vi "Vector Magnitude.vi"(1 "Z Component":dbl, 2 "Y Component":dbl, 3 "X Component":dbl) -> (0 "Magnitude":dbl)   [LabVIEW 2012]
doc: "Computes the magnitude of a two- or three-dimensional vector using the distance formula. For a two-dimensional vector simply leave the z terminal unwired."
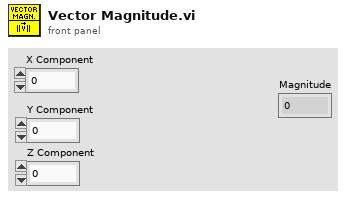
[diagram p1: front panel]
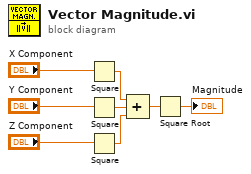
[diagram p0: block diagram]
diagram:
  n1 = Square(x="X Component") -> (x^2=w4:dbl)
  n2 = Square(x="Y Component") -> (x^2=w3:dbl)
  n3 = Square(x="Z Component") -> (x^2=w2:dbl)
  n4 = Compound Arithmetic op=ADD(w4, w3, w2) -> (w1:dbl)
  n5 = Square Root(x=w1) -> (sqrt(x)=→"Magnitude":dbl)
